vi "FeedbackDecode.vi"() -> ()   [LabVIEW 2020] (continued)
  T12 = cluster{"ExperimentDate":timestamp, "ImplantDate":timestamp, "CerebusFolder":string, "Experimenter":string, "PatientNumber":string, "DominantHand":string, "DeviceType":string, "DeviceSerial":string, "DeviceHemisphere":string, "DeviceRegion":string, "TaskType":string, "TaskComments":string, "RecordingComments":string, "GeneralObservations":string}
  T13 = typedef "FeedbackDecode_CogLoadClust.ctl" = cluster{"EEGTrigger":bool, "ConnectECG":bool, "TriggerECGwithTargets":bool, "SecondaryTask":bool, "MinTimeBetweenStimuli":dbl, "VariableTimeBetweenStimuli":dbl, "StimulusDuration":dbl, "RecordIMUwithTraining":bool, "ConnectIMU":bool}
  T14 = cluster{"[0]":u32, "[1]":u32, "[2]":u32, "[3]":u32}
  T15 = enum16{"---", "ReadMvnt", "WriteMvnt", "ReadEncode", "WriteEncode", "ReadDecode", "WriteDecode"}
  T16 = enum16{"Initialize", "Acquire Start", "Acquire Response", "Finalize"}
  T17 = enum8{"Enabled", "Disabled", "Disabled and Grayed Out"}
  T18 = enum16{"---", "Bakeoff11", "Bakeoff21", "Bakeoff31", "Bakeoff32", "LukeEmpty", "MPLEmpty", "MPLUnknown", "MPLBasic", "MPLTarg", "LukeBasic"}
  T19 = enum16{"Initialize", "Wait", "BuildInitStr", "BuildKalmanStr", "BuildStimStr", "BuildEMGStr", "GetEvent", "SendEvent", "ContIO", "LoadTrainFile", "CopyTraining", "Close"}
  T20 = cluster{"LV":cluster{"Name":string, "IP":string}, "ML":cluster{"Name":string, "IP":string}}
  T21 = enum32{"Invalid", "Standard", "Closed", "Hidden", "Minimized", "Maximized"}
  T22 = enum16{"open", "replace", "create", "open or create", "replace or create", "replace or create with confirmation"}
  T23 = enum16{"MSMS", "Bakeoff11", "Bakeoff21", "Bakeoff31", "Bakeoff32", "Bakeoff32_Ball", "Bakeoff32_Checkers", "Bakeoff32_Pen", "FragileBlock"}
  T24 = cluster{"MvntMat":dbl[][], "MvntName":string, "Tracking":enum8{"False", "True", "Mixed"}, "Radius":dbl}[]
  T25 = cluster{"Boolean 1":bool, "Boolean 2":bool, "Boolean 3":bool, "Boolean 4":bool, "Boolean 5":bool, "Boolean 6":bool, "Boolean 7":bool, "Boolean 8":bool, "Boolean 9":bool, "Boolean 10":bool, "Boolean 11":bool, "Boolean 12":bool, "Boolean 13":bool, "Boolean 14":bool, "Boolean 15":bool, "Boolean 16":bool, "Boolean 17":bool, "Boolean 18":bool, "Boolean 19":bool, "Boolean 20":bool, "Boolean 21":bool, "Boolean 22":bool, "Boolean 23":bool, "Boolean 24":bool, "Boolean 25":bool, "Boolean 26":bool, "Boolean 27":bool, "Boolean 28":bool, "Boolean 29":bool, "Boolean 30":bool, "Boolean 31":bool, "Boolean 32":bool, "Boolean 33":bool, "Boolean 34":bool, "Boolean 35":bool, "Boolean 36":bool, "Boolean 37":bool, "Boolean 38":bool, "Boolean 39":bool, "Boolean 40":bool, "Boolean 41":bool, "Boolean 42":bool, "Boolean 43":bool, "Boolean 44":bool, "Boolean 45":bool, "Boolean 46":bool, "Boolean 47":bool, "Boolean 48":bool, "Boolean 49":bool, "Boolean 50":bool, "Boolean 51":bool, "Boolean 52":bool, "Boolean 53":bool, "Boolean 54":bool, "Boolean 55":bool, "Boolean 56":bool, "Boolean 57":bool, "Boolean 58":bool, "Boolean 59":bool, "Boolean 60":bool, "Boolean 61":bool, "Boolean 62":bool, "Boolean 63":bool, "Boolean 64":bool, "Boolean 65":bool, "Boolean 66":bool, "Boolean 67":bool, "Boolean 68":bool, "Boolean 69":bool, "Boolean 70":bool, "Boolean 71":bool, "Boolean 72":bool, "Boolean 73":bool, "Boolean 74":bool, "Boolean 75":bool, "Boolean 76":bool, "Boolean 77":bool, "Boolean 78":bool, "Boolean 79":bool, "Boolean 80":bool, "Boolean 81":bool, "Boolean 82":bool, "Boolean 83":bool, "Boolean 84":bool, "Boolean 85":bool, "Boolean 86":bool, "Boolean 87":bool, "Boolean 88":bool, "Boolean 89":bool, "Boolean 90":bool, "Boolean 91":bool, "Boolean 92":bool, "Boolean 93":bool, "Boolean 94":bool, "Boolean 95":bool, "Boolean 96":bool, "Boolean 97":bool, "Boolean 98":bool, "Boolean 99":bool, "Boolean 100":bool}[]
  T26 = cluster{"[0]":dbl, "[1]":dbl, "[2]":dbl, "[3]":dbl, "[4]":dbl, "[5]":dbl, "[6]":dbl, "[7]":dbl, "[8]":dbl, "[9]":dbl, "[10]":dbl, "[11]":dbl}
  T27 = typedef "XDNodeRunTimeDep.lvlib/timing_clust.ctl" = cluster{"Expected End [f-1]":u64, "Actual End [f-1]":u64, "Finished Late? [f-1]":bool, "Expected End [i-1]":u64, "Actual End [i-1]":u64, "Finished Late? [i-1]":bool, "Expected Start [i]":u64, "Actual Start [i]":u64, "Expected Start [f]":u64, "Actual Start [f]":u64, "Source Name":string, "Structure Name":string, "Period":i64, "Deadline":i64, "Offset":i64, "Start":i64, "Priority":i32, "Timeout":i32, "Mode":T28, "Wakeup Reason":T29, "Error":errorcluster, "Source Type":string, "Secondary Source Type":string, "Global End Time":u64, "Global Start Time":u64, "Frame Duration":u64, "Iteration Duration":u64, "Assigned CPU":i32, "I/O Scan Engine Mode":u32}
  T28 = typedef "XDNodeRunTimeDep.lvlib/nitl_modes.ctl" = enum32{"No Change", "Process missed periods, maintain original phase", "Discard missed periods, maintain original phase", "Process missed periods, ignore original phase", "Discard missed periods, ignore original phase"}
  T29 = typedef "XDNodeRunTimeDep.lvlib/wakeup.ctl" = enum32{"Normal", "Aborted", "Asynchronous wakeup", "Timing source error", "Timed loop error", "Timeout"}
  T30 = enum16{"MSMS", "BakeOff1", "BakeOff2", "BakeOff3"}
  T31 = typedef "LVPositionTypeDef.ctl" = cluster{"Left":i32, "Top":i32}
  T32 = typedef "LVBoundsTypeDef.ctl" = cluster{"Width":u32, "Height":u32}
  T33 = cluster{cluster{"[0]":u32, "[1]":u32, "[2]":u32, "[3]":u32}, "HMSize":cluster{"NumCol":dbl, "NumRows":dbl}}
  T34 = cluster{"Left":i32, "Top":i32, "Width":u32, "Height":u32}
  T35 = cluster{"Name":string, "Type":string, "ID":string, "Num":string, "COM":dbl[], "Offset":dbl[], "RotationAxis":dbl[], "OrientationMatrix":dbl[][], "MinAngle":dbl, "MaxAngle":dbl, "InboardID":string, "InboardNum":string, "InboardCOM":dbl[], "OutboardID":string, "OutboardNum":string, "OutboardCOM":dbl[]}[]
  T36 = cluster{"ModelName":string, "Value":dbl[][], "CompNames":string[]}
  T37 = enum16{"Off", "Training", "Decode", "COB", "LEAP"}
  T38 = cluster{"ContMvntVal[0]":dbl, "ContMvntVal[1]":dbl, "ContMvntVal[2]":dbl, "ContMvntVal[3]":dbl, "ContMvntVal[4]":dbl, "ContMvntVal[5]":dbl, "ContMvntVal[6]":dbl, "ContMvntVal[7]":dbl, "ContMvntVal[8]":dbl, "ContMvntVal[9]":dbl, "ContMvntVal[10]":dbl, "ContMvntVal[11]":dbl}
  T39 = cluster{"ContTargetVal[0]":dbl, "ContTargetVal[1]":dbl, "ContTargetVal[2]":dbl, "ContTargetVal[3]":dbl, "ContTargetVal[4]":dbl, "ContTargetVal[5]":dbl, "ContTargetVal[6]":dbl, "ContTargetVal[7]":dbl, "ContTargetVal[8]":dbl, "ContTargetVal[9]":dbl, "ContTargetVal[10]":dbl, "ContTargetVal[11]":dbl}
  T40 = cluster{"LoopTimings":cluster{"MLCalcTime":dbl, "MLTotalTime":dbl}, "Kalman":cluster{"Thumb":dbl, "Index":dbl, "Middle":dbl, "Ring":dbl, "Little":dbl, "ThumbInt":dbl, "IndexInt":dbl, "RingInt":dbl, "LittleInt":dbl, "Wrist":dbl, "WristYaw":dbl, "WristRoll":dbl}, "Kinematics":cluster{"Thumb":dbl, "Index":dbl, "Middle":dbl, "Ring":dbl, "Little":dbl, "ThumbInt":dbl, "IndexInt":dbl, "RingInt":dbl, "LittleInt":dbl, "Wrist":dbl, "WristYaw":dbl, "WristRoll":dbl}, "ElectRates":dbl[], "SelWfs":dbl[][], "TrainCnt":dbl, "EMGPwr":dbl[], "SelData":cluster{dbl, dbl, "RasterOut":dbl[]}[], "SelRate":cluster{"CurIdx":dbl, dbl, "RasterOut":dbl[]}[], "SelKin":cluster{dbl, dbl, "RasterOut":dbl[]}[], "NIPTime":dbl, "VREID":i16, "StimWf":dbl[], "RawDecodeOutput":dbl[], "TASKA IR sensors":dbl[], "TASKA baro sensors":dbl[]}
  T41 = cluster{"Thumb":dbl, "Index":dbl, "Middle":dbl, "Ring":dbl, "Little":dbl, "ThumbInt":dbl, "IndexInt":dbl, "RingInt":dbl, "LittleInt":dbl, "Wrist":dbl, "WristYaw":dbl, "WristRoll":dbl}
  T42 = cluster{"Delay":dbl, "Rise":dbl, "Hold":dbl, "Trial":dbl}
  T43 = enum16{"Position", "Latching", "Leaky", "Velocity"}[]
  T44 = enum16{"Standard", "Mean", "Refit", "LinSVReg", "NonLinSVReg", "PCA", "DWPRR", "AdaptKF", "NN", "NN_python", "AdaptKF2", "KF_Short_Goal"}
  T45 = typedef "LVPoint32TypeDef.ctl" = cluster{"Horizontal":i32, "Vertical":i32}
  T46 = cluster{"KGain":sgl[][], "KMvnts":cluster{"Thumb":bool, "Index":bool, "Middle":bool, "Ring":bool, "Little":bool, "ThumbInt":bool, "IndexInt":bool, "RingInt":bool, "LittleInt":bool, "WristPitch":bool, "WristYaw":bool, "WristRoll":bool}, "KThresh":sgl[][], "CtrlMode":enum16{"Position", "Latching", "Leaky", "Velocity"}[], "CtrlSpd":sgl[]}
  T47 = enum16{"RMS Single", "RMS All", "RMS Auto", "Volt Single", "Volt All"}
  T48 = cluster{"[0]":bool, "[1]":bool, "[2]":bool, "[3]":bool, "[4]":bool, "[5]":bool, "[6]":bool, "[7]":bool, "[8]":bool, "[9]":bool, "[10]":bool, "[11]":bool, "[12]":bool, "[13]":bool, "[14]":bool, "[15]":bool, "[16]":bool, "[17]":bool, "[18]":bool, "[19]":bool, "[20]":bool, "[21]":bool, "[22]":bool, "[23]":bool, "[24]":bool, "[25]":bool, "[26]":bool, "[27]":bool, "[28]":bool, "[29]":bool, "[30]":bool, "[31]":bool, "[32]":bool, "[33]":bool, "[34]":bool, "[35]":bool, "[36]":bool, "[37]":bool, "[38]":bool, "[39]":bool, "[40]":bool, "[41]":bool, "[42]":bool, "[43]":bool, "[44]":bool, "[45]":bool, "[46]":bool, "[47]":bool, "[48]":bool, "[49]":bool, "[50]":bool, "[51]":bool, "[52]":bool, "[53]":bool, "[54]":bool, "[55]":bool, "[56]":bool, "[57]":bool, "[58]":bool, "[59]":bool, "[60]":bool, "[61]":bool, "[62]":bool, "[63]":bool, "[64]":bool, "[65]":bool, "[66]":bool, "[67]":bool, "[68]":bool, "[69]":bool, "[70]":bool, "[71]":bool, "[72]":bool, "[73]":bool, "[74]":bool, "[75]":bool, "[76]":bool, "[77]":bool, "[78]":bool, "[79]":bool, "[80]":bool, "[81]":bool, "[82]":bool, "[83]":bool, "[84]":bool, "[85]":bool, "[86]":bool, "[87]":bool, "[88]":bool, "[89]":bool, "[90]":bool, "[91]":bool, "[92]":bool, "[93]":bool, "[94]":bool, "[95]":bool, "[96]":bool, "[97]":bool, "[98]":bool, "[99]":bool}
  T49 = cluster{"[0]":bool, "[1]":bool, "[2]":bool, "[3]":bool, "[4]":bool, "[5]":bool, "[6]":bool, "[7]":bool, "[8]":bool, "[9]":bool, "[10]":bool, "[11]":bool, "[12]":bool, "[13]":bool, "[14]":bool, "[15]":bool, "[16]":bool, "[17]":bool, "[18]":bool, "[19]":bool, "[20]":bool, "[21]":bool, "[22]":bool, "[23]":bool, "[24]":bool, "[25]":bool, "[26]":bool, "[27]":bool, "[28]":bool, "[29]":bool, "[30]":bool, "[31]":bool, "[32]":bool, "[33]":bool, "[34]":bool, "[35]":bool, "[36]":bool, "[37]":bool, "[38]":bool, "[39]":bool, "[40]":bool, "[41]":bool, "[42]":bool, "[43]":bool, "[44]":bool, "[45]":bool, "[46]":bool, "[47]":bool, "[48]":bool, "[49]":bool, "[50]":bool, "[51]":bool, "[52]":bool, "[53]":bool, "[54]":bool, "[55]":bool, "[56]":bool, "[57]":bool, "[58]":bool, "[59]":bool, "[60]":bool, "[61]":bool, "[62]":bool, "[63]":bool, "[64]":bool, "[65]":bool, "[66]":bool, "[67]":bool, "[68]":bool, "[69]":bool, "[70]":bool, "[71]":bool, "[72]":bool, "[73]":bool, "[74]":bool, "[75]":bool, "[76]":bool, "[77]":bool, "[78]":bool, "[79]":bool}
  T50 = enum16{"Position", "Latching", "Leaky", "Velocity"}
  T51 = cluster{"Shift":bool, "Ctrl":bool, "Alt":bool, "Cmd":bool, "Opt":bool}
  T52 = cluster{"Region":bool, "Receptor":bool, "Electrode":bool, "Min Amp":bool, "Max Amp":bool, "Min Freq":bool, "Max Freq":bool, "Duration":bool}
  T53 = typedef "eventvkey.ctl" = enum16{"ASCII", "Enter", "Return", "Shift", "Ctrl", "Alt", "Cmd", "Opt", "Caps", "NumLock", "Clear", "Break", "Up", "Down", "Left", "Right", "Insert", "Delete", "Home", "End", "PageUp", "PageDown", "Escape", "Help", "Pause", "ScrollLock", "F1", "F2", "F3", "F4", "F5", "F6", "F7", "F8", "F9", "F10", "F11", "F12", "F13", "F14", "F15", "F16", "F17", "F18", "F19", "F20", "F21", "F22", "F23", "F24", "Play", "VolumeUp", "VolumeDown", "Mute", "Two Byte Char"}
  T54 = cluster{"Boolean 1":bool, "Boolean 2":bool, "Boolean 3":bool, "Boolean 4":bool, "Boolean 5":bool, "Boolean 6":bool, "Boolean 7":bool, "Boolean 8":bool, "Boolean 9":bool, "Boolean 10":bool, "Boolean 11":bool, "Boolean 12":bool, "Boolean 13":bool, "Boolean 14":bool, "Boolean 15":bool, "Boolean 16":bool, "Boolean 17":bool, "Boolean 18":bool, "Boolean 19":bool, "Boolean 20":bool, "Boolean 21":bool, "Boolean 22":bool, "Boolean 23":bool, "Boolean 24":bool, "Boolean 25":bool, "Boolean 26":bool, "Boolean 27":bool, "Boolean 28":bool, "Boolean 29":bool, "Boolean 30":bool, "Boolean 31":bool, "Boolean 32":bool, "Boolean 33":bool, "Boolean 34":bool, "Boolean 35":bool, "Boolean 36":bool, "Boolean 37":bool, "Boolean 38":bool, "Boolean 39":bool, "Boolean 40":bool, "Boolean 41":bool, "Boolean 42":bool, "Boolean 43":bool, "Boolean 44":bool, "Boolean 45":bool, "Boolean 46":bool, "Boolean 47":bool, "Boolean 48":bool, "Boolean 49":bool, "Boolean 50":bool, "Boolean 51":bool, "Boolean 52":bool, "Boolean 53":bool, "Boolean 54":bool, "Boolean 55":bool, "Boolean 56":bool, "Boolean 57":bool, "Boolean 58":bool, "Boolean 59":bool, "Boolean 60":bool, "Boolean 61":bool, "Boolean 62":bool, "Boolean 63":bool, "Boolean 64":bool, "Boolean 65":bool, "Boolean 66":bool, "Boolean 67":bool, "Boolean 68":bool, "Boolean 69":bool, "Boolean 70":bool, "Boolean 71":bool, "Boolean 72":bool, "Boolean 73":bool, "Boolean 74":bool, "Boolean 75":bool, "Boolean 76":bool, "Boolean 77":bool, "Boolean 78":bool, "Boolean 79":bool, "Boolean 80":bool, "Boolean 81":bool, "Boolean 82":bool, "Boolean 83":bool, "Boolean 84":bool, "Boolean 85":bool, "Boolean 86":bool, "Boolean 87":bool, "Boolean 88":bool, "Boolean 89":bool, "Boolean 90":bool, "Boolean 91":bool, "Boolean 92":bool, "Boolean 93":bool, "Boolean 94":bool, "Boolean 95":bool, "Boolean 96":bool, "Boolean 97":bool, "Boolean 98":bool, "Boolean 99":bool, "Boolean 100":bool}
  T55 = cluster{"[0]":bool, "[1]":bool, "[2]":bool, "[3]":bool, "[4]":bool, "[5]":bool, "[6]":bool, "[7]":bool, "[8]":bool, "[9]":bool, "[10]":bool, "[11]":bool, "[12]":bool, "[13]":bool, "[14]":bool, "[15]":bool, "[16]":bool, "[17]":bool, "[18]":bool, "[19]":bool, "[20]":bool, "[21]":bool, "[22]":bool, "[23]":bool, "[24]":bool, "[25]":bool, "[26]":bool, "[27]":bool, "[28]":bool, "[29]":bool, "[30]":bool, "[31]":bool, "[32]":bool, "[33]":bool, "[34]":bool, "[35]":bool, "[36]":bool, "[37]":bool, "[38]":bool, "[39]":bool, "[40]":bool, "[41]":bool, "[42]":bool, "[43]":bool, "[44]":bool, "[45]":bool, "[46]":bool, "[47]":bool, "[48]":bool, "[49]":bool, "[50]":bool, "[51]":bool, "[52]":bool, "[53]":bool, "[54]":bool, "[55]":bool, "[56]":bool, "[57]":bool, "[58]":bool, "[59]":bool, "[60]":bool, "[61]":bool, "[62]":bool, "[63]":bool, "[64]":bool, "[65]":bool, "[66]":bool, "[67]":bool, "[68]":bool, "[69]":bool, "[70]":bool, "[71]":bool, "[72]":bool, "[73]":bool, "[74]":bool, "[75]":bool, "[76]":bool, "[77]":bool, "[78]":bool, "[79]":bool, "[80]":bool, "[81]":bool, "[82]":bool, "[83]":bool, "[84]":bool, "[85]":bool, "[86]":bool, "[87]":bool, "[88]":bool, "[89]":bool, "[90]":bool, "[91]":bool, "[92]":bool, "[93]":bool, "[94]":bool, "[95]":bool, "[96]":bool, "[97]":bool, "[98]":bool, "[99]":bool}[]
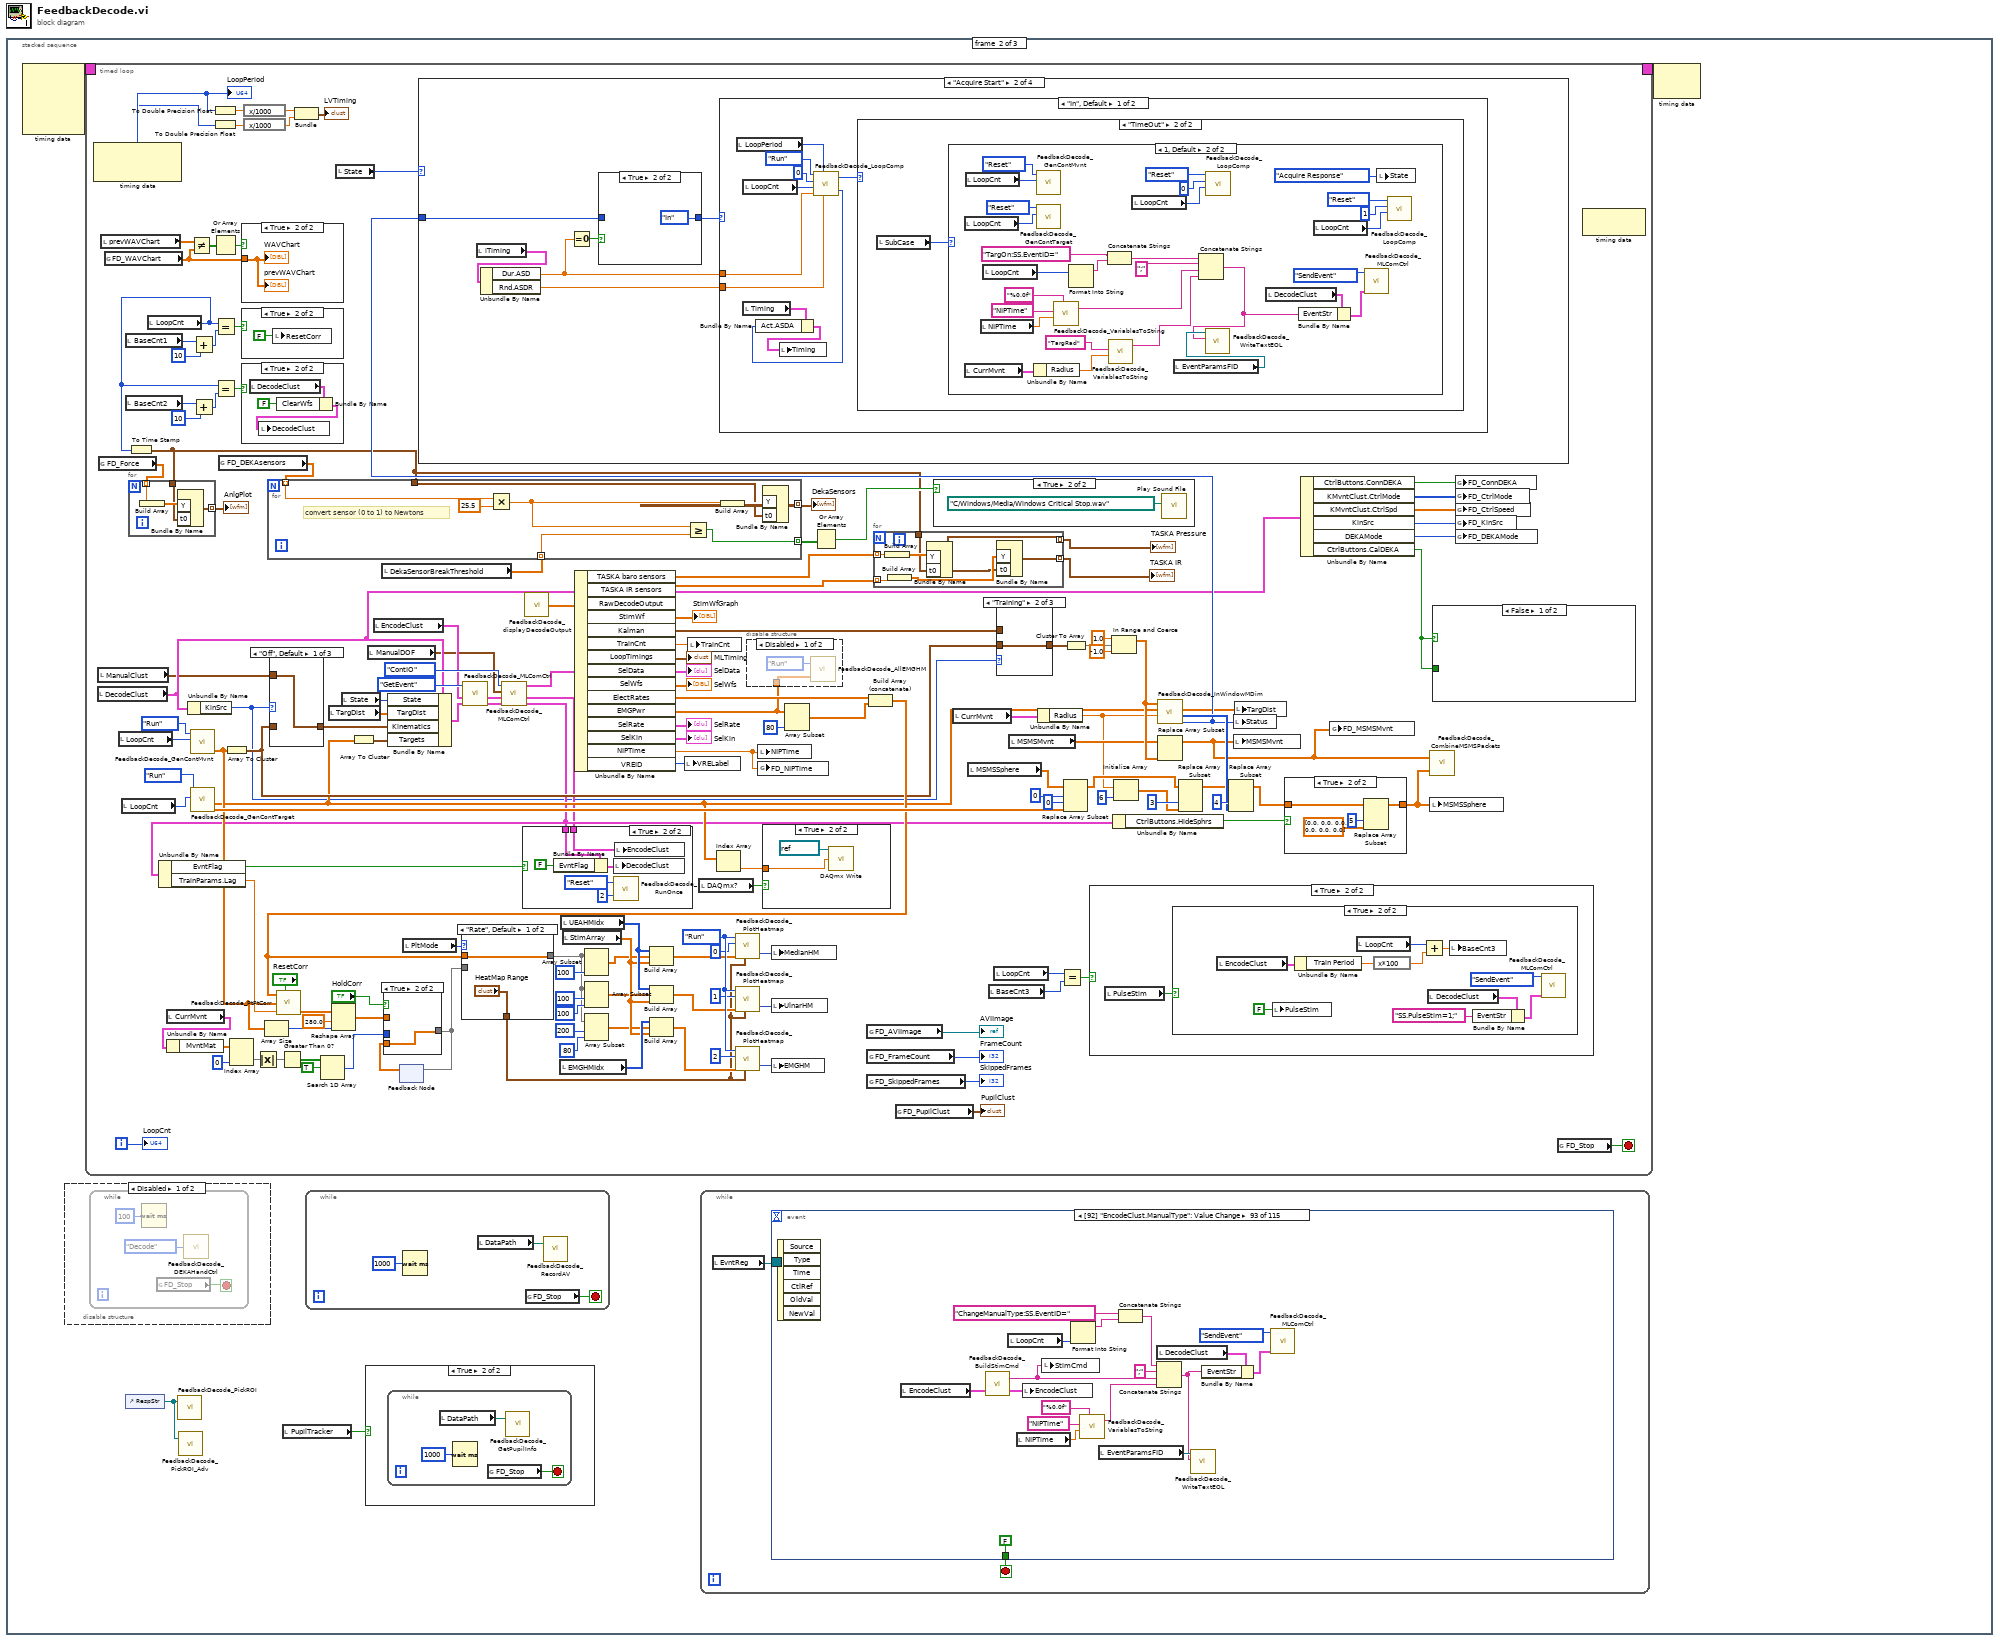
[diagram p0: block diagram]
diagram:
  n1 = stacked-sequence {
    frame #0 {
      n2 = stacked-sequence {
        frame #0 {
          w45 = FALSE ("Finished")
          w52 = 0.0  # MvntEvnt
          w68 = u64 0 ("BaseCnt1")
          w155 = enum16{"Initialize", "Reset", "Run"}."Initialize" ("Mode")
          w141 = "" ("TrialTypeStr")
          w122 = path "Z:/Shared drives/CNI/General/Databases/PatientDatabase.udl" ("DatabaseUDL")
          # "Is shared enabled?"
          # "TASKA"
          # "for analog sensors"
          n3 = local write "TASKASharedControlBeta"(0.0 ("TASKASharedControlBeta")) -> ()
          n4 = local write "Beta Mode"("Fixed" ("Beta Mode")) -> ()
          n5 = local write "Computer Goal"("Close" ("Computer Goal")) -> ()
          n6 = local write "TASKA Shared Control"(FALSE ("TASKA Shared Control")) -> ()
          n7 = property on="MedianHM" class="Pict"() -> ("Position"=w119:T31, "Draw Area Size"=w118:T32)  [unwired: 2 in, 2 out]
          n8 = property on="UlnarHM" class="Pict"() -> ("Position"=w114:T31, "Draw Area Size"=w115:T32)  [unwired: 2 in, 2 out]
          n9 = property on="EMGHM" class="Pict"() -> ("Position"=w100:T31, "Draw Area Size"=w99:T32)  [unwired: 2 in, 2 out]
          n10 = Initialize Array(0.0 ("element"), 496 ("dimension size")) -> (w54:dbl[])
          n11 = Cluster To Array(cluster=w119) -> (array=w148:i32[])
          n12 = Cluster To Array(cluster=w118) -> (array=w149:u32[])
          n13 = Cluster To Array(cluster=w114) -> (array=w113:i32[])
          n14 = Cluster To Array(cluster=w115) -> (array=w112:u32[])
          n15 = Cluster To Array(cluster=w100) -> (array=w101:i32[])
          n16 = Cluster To Array(cluster=w99) -> (array=w102:u32[])
          n17 = call "FeedbackDecode_AllEMGHM.vi"("Intensities"=w54, "Mode"=enum16{"Initialize", "Run"}."Initialize") -> ()  [unwired: 2 in]
          n18 = property on="Finished" class="Bool (strict)"("DisabledEnum"=T17."Disabled and Grayed Out" ("Disabled"), "Value"=w45, "Blinking"=w45) -> ()  [unwired: 2 in, 2 out]
          n19 = Build Array (concatenate)(w148, w149) -> (w150:u32[])
          n20 = Build Array (concatenate)(w113, w112) -> (w111:u32[])
          n21 = Build Array (concatenate)(w101, w102) -> (w103:u32[])
          n22 = mathscript code="GridArray = reshape(rot90(reshape(1:100,10,10),-1),1,100);"() -> ("GridArray"=→"UEAHMIdx":i32[])  [unwired: 1 in, 1 out]
          n23 = property on="ParamsTable" class="Arr (strict)"() -> ("Index Values"=w81:u32[], "Left"=w73:i32, "Width"=w72:u32)  [unwired: 2 in, 2 out]
          n24 = Array To Cluster(array=w150) -> (cluster=w151:T14)
          "MedianPos" <- w151
          n25 = Array To Cluster(array=w111) -> (cluster=w107:T14)
          "UlnarPos" <- w107
          n26 = Array To Cluster(array=w103) -> (cluster=w98:T14)
          "EMGPos" <- w98
          n27 = for {
            N: 2 -> [_]
            tunnel: [w180] -> w43 mode=indexing
            i -> [w179]
            n28 = case shown="0, Default" w179 {
              tunnel: [w181 w185] -> w180
              frame 0, Default {
                n29 = vi-ref "FeedbackDecode_PickROI.vi"() -> (w184:refnum<vi>)
                n30 = invoke class="VI" method="FP.Open"(reference=w184, "Activate"=TRUE ("Activate?"), "State"=T21."Hidden") -> (reference out=w181:refnum<vi>)  [unwired: 2 in, 4 out]
              }
              frame 1 {
                n31 = vi-ref "FeedbackDecode_PickROI_Adv.vi"() -> (w188:refnum<vi>)
                n32 = invoke class="VI" method="FP.Open"(reference=w188, "Activate"=TRUE ("Activate?"), "State"=T21."Hidden") -> (reference out=w185:refnum<vi>)  [unwired: 2 in, 4 out]
              }
            }
          }
          "RespRefArray" <- w43
          n33 = stacked-sequence {
            frame #0 {
              w171 = FALSE ("TASKA Reset Success")
              n34 = local write "TASKA Reset Success"(w171) -> ()
              n35 = local write "TASKA Reset Break"(w171) -> ()
              n36 = local write "TASKA Timer"(w171) -> ()
            }
            frame #1 {
              n37 = property on="TASKA Timer" class="Bool (strict)"("DisabledEnum"=T17."Enabled" ("Disabled")) -> ()  [unwired: 2 in, 2 out]
            }
          }
          n38 = Bundle(w151, "HMSize"="HMSize") -> (w152:T33)  [unwired: 1 in]
          n39 = Bundle(w107, "HMSize"="HMSize") -> (w108:T33)  [unwired: 1 in]
          n40 = Bundle(w98, "HMSize"="HMSize") -> (w106:T33)  [unwired: 1 in]
          n41 = call "FeedbackDecode_PlotHeatmap.vi"("InitCluster"=w152, "Instance"=0, "Mode"=enum16{"Initialize", "Run", "Mouse"}."Initialize") -> ("Pic"=→"MedianHM":picture, "CurrPos"=w92:i32)  [unwired: 3 in]
          "SelElect" <- w92
          n42 = call "FeedbackDecode_PlotHeatmap.vi"("InitCluster"=w108, "Instance"=1, "Mode"=enum16{"Initialize", "Run", "Mouse"}."Initialize") -> ("Pic"=→"UlnarHM":picture)  [unwired: 3 in, 1 out]
          n43 = call "FeedbackDecode_PlotHeatmap.vi"("InitCluster"=w106, "Instance"=2, "Mode"=enum16{"Initialize", "Run", "Mouse"}."Initialize") -> ("Pic"=→"EMGHM":picture)  [unwired: 3 in, 1 out]
          n44 = property on="Sel" class="Arr (strict)"("Index Values"=w81) -> ()  [unwired: 2 in, 2 out]
          n45 = Bundle("Left"=w73, "Width"=w72) -> (→"ParamsTableLoc":cluster{"Left":i32, "Width":u32})  [unwired: 1 in]
          n46 = disable-structure shown="Disabled" {
            frame Disabled {
              n47 = vi-ref "FeedbackDecode_MSMS2DEKA.vi"() -> (w178:refnum<vi>)
              n48 = invoke class="VI" method="FP.Open"(reference=w178, "Activate"=FALSE ("Activate?"), "State"=T21."Minimized") -> ()  [unwired: 2 in, 5 out]
            }
            frame Enabled {
            }
          }
          n49 = property class="VI"() -> ("Name"=→"TaskType":string)  [unwired: 2 in, 2 out]
          n50 = property on="KUEA" class="Clust (strict)"() -> ("Left"=w166:i32, "Top"=w165:i32, "Width"=w164:u32, "Height"=w163:u32)  [unwired: 2 in, 2 out]
          n51 = for {
            N: 80 -> [_]
            tunnel: [w192] -> w96 mode=indexing
            i -> [w193]
            n52 = Increment(x=w193) -> (x+1=w192:i32)
          }
          "EMGHMIdx" <- w96
          n53 = Initialize Array(0.0 ("element"), 100 ("dimension size")) -> (→"StimArray":dbl[])
          n54 = Bundle("Left"=w166, "Top"=w165, "Width"=w164, "Height"=w163) -> (w162:T34)  [unwired: 1 in]
          "HoverPicPos" <- w162
          n55 = call <vilib>:"Application Directory.vi"() -> ("Application Directory"=w2:path)
          n56 = call <vilib>:"Check if File or Folder Exists.vi"("path"=path "D:/") -> ("file or folder exists?"=w21:bool)  [unwired: 8 in, 2 out]
          n57 = vi-ref "FeedbackDecode_PlaySound.vi"() -> (w157:refnum<vi>)
          n58 = disable-structure shown="Disabled" {
            frame Disabled {
              n59 = vi-ref "FeedbackDecode_AllEMGHM.vi"() -> (w189:refnum<vi>)
              n60 = invoke class="VI" method="FP.Open"(reference=w189, "Activate"=FALSE ("Activate?"), "State"=T21."Minimized") -> ()  [unwired: 2 in, 5 out]
            }
            frame Enabled {
            }
          }
          n61 = Build Path(base path=w2, name or relative path="resources") -> (appended path=w1:path)
          "ResourcesDir" <- w1
          n62 = Build Path(base path=w2, name or relative path="build") -> (appended path=w13:path)
          "BuildDir" <- w13
          n63 = call "FeedbackDecode_HoverElect.vi"("Border"=2.0, "PicPos"=w162, "Mode"=enum16{"Initialize", "Run"}."Initialize") -> ("Elect"=w143:i32)  [unwired: 3 in, 1 out]
          n64 = property class="VI"(reference=w157) -> ("Name"=w156:string)  [unwired: 1 in, 2 out]
          n65 = Select(t=path "D:/FeedbackDecode", s=w21, f=path "C:/Data/FeedbackDecode" ("path")) -> (s? t:f=w17:path)
          "DataDir" <- w17
          n66 = global write "FeedbackDecode_Globals.vi" "FD_ResourcesDir"(w1) -> ()
          n67 = Unbundle By Name("DecodeClust") -> ("NumComp"=w26:enum16{"1 Computer", "2 Computers"})
          n68 = Path To String(path=w13) -> (string=w15:string)
          n69 = Path To String(path=w17) -> (string=w19:string)
          n70 = Unbundle By Name("MvntBuilder") -> ("Mode"=w36:enum16{"Selected", "Block", "Random"}, "NTrials"=w39:dbl, "MvntList"=w40:T24)
          n71 = property on="MvntList" class="Arr (strict)"() -> ("Index Values"=w42:u32[])  [unwired: 2 in, 2 out]
          n72 = Open VI Reference(type specifier VI Refnum (for type only)=refnum<vi> refnum ("application reference (local)"), vi path=w156, options=128) -> (vi reference=→"PSRef":refnum<vi>)  [unwired: 3 in, 1 out]
          n73 = Unbundle By Name("MvntBuilder") -> ("TargParams.Radius"=w87:dbl)
          n74 = Search and Replace String(input string=w15, search string=":", replace string="@" ("replace string (\"\")")) -> (result string=w12:string)  [unwired: 5 in, 3 out]
          n75 = Search and Replace String(input string=w19, search string=":", replace string="@" ("replace string (\"\")")) -> (result string=w11:string)  [unwired: 5 in, 3 out]
          n76 = case shown="\"1 Computer\"" w26 {
            tunnel: [T20 {"LV"={"Name"="PNILABVIEW", "IP"="155.100.90.215"}, "ML"={"Name"="PNIMATLAB", "IP"="155.100.90.185"}} ("CompID") T20 {"LV"={"Name"="PNILABVIEW", "IP"="127.0.0.1"}, "ML"={"Name"="PNIMATLAB", "IP"="127.0.0.2"}} ("CompID")] -> w25
            frame "2 Computers", Default {
            }
            frame "1 Computer" {
            }
          }
          n77 = Array Size(array=w40) -> (size(s)=w41:i32)
          n78 = Index Array(array=w42) -> (element=w38:u32)  [unwired: 1 in]
          n79 = call "FeedbackDecode_GenRandBlockIdxs2.vi"("Mode"=w36, "Reset"=TRUE, "NumTrials"=w39, "NumIdxs"=w41, "CurrIdx"=w38) -> ("Perc"=w34:dbl)  [unwired: 1 out]
          n80 = Initialize Array(0.0 ("element"), 2 ("dimension size"), 12 ("dimension size")) -> (w77:dbl[][])
          n81 = Bundle By Name(cluster="MvntBuilder", "PercTrials"=w34) -> (w33:T6)
          n82 = call "FeedbackDecode_RunOnce.vi"("Instance"=0, "Mode"=enum16{"Reset", "Run"}."Reset") -> ()  [unwired: 1 out]
          n83 = Bundle By Name(cluster="DecodeClust", "BuildDir"=w12, "DataDir"=w11, "TrainParams.TargRad"=w87, "DataFolder"="00000000-000000", "SelElect"=w92, "CompID"=w25, "HoverElect"=w143, "KinSrc"=enum16{"Off", "Training", "Decode", "COB"}."Off", "TrialCnt"=w77, "KDFFile"="") -> (w84:T5)
          n84 = Unbundle By Name(w25) -> ("LV.IP"=→"LVIP":string, "ML.IP"=→"MLIP":string)
          n85 = local write "MvntBuilder"(w33) -> ()
          n86 = call "FeedbackDecode_RunOnce.vi"("Instance"=1, "Mode"=enum16{"Reset", "Run"}."Reset") -> ()  [unwired: 1 out]
          n87 = call "FeedbackDecode_RunOnce.vi"("Instance"=2, "Mode"=enum16{"Reset", "Run"}."Reset") -> ()  [unwired: 1 out]
          n88 = global write "FeedbackDecode_Globals.vi" "FD_Stop"(FALSE ("EnablePtCtrl")) -> ()
          n89 = call "FeedbackDecode_MLComCtrl.vi"("CognitiveLoadIn"="CognitiveLoad", "DecodeClustIn"=w84, "EncodeClustIn"="EncodeClust", "Mode"=T19."Initialize") -> ("DecodeClustOut"=w32:T5, "EncodeClustOut"=w82:T9, "CognitiveLoadOut"=w4:T13)  [unwired: 4 in, 1 out]
          n90 = property class="DAQmx System"() -> ("DevNames"=w30:tag[])  [unwired: 2 in, 2 out]
          n91 = Unbundle By Name(w32) -> ("RasterWin"=w88:dbl)
          n92 = Unbundle By Name(w32) -> ("*Prosthesis"=w58:enum16{"MaleRight", "MaleLeft"})
          n93 = Create User Event(user event datatype=w52) -> (user event=w51:refnum<user-event>)  [unwired: 1 in, 1 out]
          "MvntEvnt" <- w51
          n94 = local write "EncodeClust"(w82) -> ()
          n95 = local write "CognitiveLoad"(w4) -> ()
          n96 = local write "DecodeClust"(w32) -> ()
          n97 = register-events(w51) -> (reference out=→"EvntReg":refnum<event-registration>)  [unwired: 2 in, 1 out]
          n98 = Divide(x=w88, y=0.033) -> (x/y=w85:dbl)
          n99 = Empty Array?(array=w30) -> (empty?=w29:bool)
          n100 = Format Into String(w58) -> (resulting string=w135:string)  [unwired: 3 in, 1 out]
          n101 = Multiply(x=2.0, y=w85) -> (x*y=w86:dbl)
          n102 = Not(x=w29) -> (.not. x?=→"DAQmx?":bool)
          n103 = property on="SelData" class="WFGraph (strict)"("XScale.Maximum"=w86) -> ()  [unwired: 2 in, 2 out]
          n104 = property on="SelRate" class="WFGraph (strict)"("XScale.Maximum"=w85) -> ()  [unwired: 2 in, 2 out]
          n105 = property on="SelKin" class="WFGraph (strict)"("XScale.Maximum"=w85) -> ()  [unwired: 2 in, 2 out]
          n106 = case shown="False" w29 {
            frame False {
              n107 = call <vilib>:"DAQmx Start Task.vi"("task/channels in"=refnum<k21> "AO0") -> ()  [unwired: 13 in, 2 out]
            }
            frame True {
            }
          }
          n108 = Concatenate Strings("Z:\\Shared drives\\CNI\\General\\MSMS\\Scenarios\\", w135, "\\Model\\Prostheses\\prosthesis.xml") -> (w137:string)
          n109 = String To Path(string=w137) -> (path=w138:path)
          "XMLFile" <- w138
          n110 = call "FeedbackDecode_ParseMSMSXML.vi"("XMLFile"=w138) -> ("ComponentArray"=w132:T35)
          n111 = call "FeedbackDecode_UpdateDatabase.vi"("CallType"=enum16{"Initialize", "Save", "Load"}."Initialize", "DatabaseUDL"=w122) -> ("ExperimentDatesSorted"=w124:string[])  [unwired: 2 in, 2 out]
          n112 = call "FeedbackDecode_LoadMSMSParams.vi"("XMLFile"=w138) -> ("ModelParams"=w133:T36)  [unwired: 1 in]
          n113 = call "FeedbackDecode_SendMSMSPacket.vi"("CompArrayIn"=w132, "Mode"=enum16{"Initialize", "Run", "Close"}."Initialize") -> ()  [unwired: 5 in]
          n114 = property on="RecordSel" class="CmbBox"("Text.Text"="", "Strings[]"=w124) -> ()  [unwired: 2 in, 2 out]
          n115 = call "FeedbackDecode_BuildMSMSMvnt.vi"("CompArray"=w132, "ModelParams"=w133, "Mode"=enum16{"Initialize", "Run"}."Initialize") -> ()  [unwired: 4 in, 3 out]
          n116 = call "FeedbackDecode_GenContTarget.vi"("Mode"=w155) -> ()  [unwired: 5 in, 4 out]
          n117 = call "FeedbackDecode_GenContMvnt.vi"("Mode"=w155) -> ()  [unwired: 5 in, 3 out]
          n118 = call "FeedbackDecode_BuildMSMSSphere.vi"("CompArray"=w132, "ModelParams"=w133, "Mode"=enum16{"Initialize", "Run"}."Initialize") -> ()  [unwired: 4 in, 3 out]
          "State" <- T16."Initialize" ("Current State")
          "BaseCnt1" <- w68
          "TrialParameters" <- w141
          "DatabaseUDL" <- w122
          "TaskParameters" <- w141
          "Outcome" <- enum16{"---", "Success", "Failure"}."---" ("Outcome")
          "TrialArray" <- string[] [] ("TrialArray")
          "PrevIdx" <- 0.0 ("PrevIdx")
          "BaseCnt2" <- w68
          "TrainCnt" <- 0.0 ("TrainCnt")
          "Status" <- enum16{"In", "Out"}."Out" ("Status")
          "FileIO" <- T15."---" ("FileIO")
          "TargDist" <- dbl[] [0.0, 0.0, 0.0, 0.0, 0.0, 0.0] ("TargDist")
          "iTiming" <- "Timing"
          "NIPTime" <- 0.0 ("TrainCnt")
          "VRELabel" <- T18."---" ("VRELabel")
          "BaseCnt3" <- -inf
          "PulseStim" <- FALSE ("PulseStim")
          "RespStr" <- ""
          "StimCmd" <- ""
          "SelTog" <- FALSE ("SelTog")
          "StimTog" <- FALSE ("StimTog")
          "CurrMvnt" <- T1 {"MvntMat"=[], "MvntName"="", "Tracking"=enum."False", "Radius"=0.15} ("CurrMvnt")
        }
        frame #1 {
          # "Open Trellis if it is not already running"
          n119 = call <vilib>:"System Exec.vi"("command line"="powershell -inputformat none -command get-process -name Trellis") -> ("error out"=w242:errorcluster, "standard output"=w244:string)  [unwired: 7 in, 2 out]
          n120 = Empty String/Path?(string/path=w244) -> (empty?=w243:bool)
          n121 = case shown="True" w243 {
            tunnel: [w246 w248] -> w241
            tunnel: w242 -> [w246 w247]
            frame False {
            }
            frame True {
              n122 = Path To String(path=path "C:/Program Files (x86)/Ripple/Trellis/Apps/Trellis/bin/start_Trellis.bat") -> (string=w251:string)
              n123 = call <vilib>:"System Exec.vi"("wait until completion? (T)"=FALSE, "error in (no error)"=w247, "working directory"=path "C:/Program Files (x86)/Ripple/Trellis/Apps/Trellis/bin", "command line"=w251) -> ("error out"=w248:errorcluster)  [unwired: 4 in, 3 out]
            }
          }
          n124 = case shown="No Error" w241 {
            tunnel: w241 -> [_ w254]
            frame No Error {
              n125 = One Button Dialog(message="Load Trellis config file, enable appropriate channels for saving to disk, set file save directory to \"D:\\\", and make sure digital triggering is enabled.\n\nDigital Triggering...\nStart: Parallel (0x007F; 0x0011)\nStop: Parallel (0x007F; 0x0012) ") -> ()  [unwired: 1 in, 1 out]
            }
            frame Error {
              n126 = call <vilib>:"Simple Error Handler.vi"("error in (no error)"=w254) -> ()  [unwired: 4 in, 5 out]
            }
          }
        }
        frame #2 {
          n127 = call "FeedbackDecode_CheckPupilConnection.vi"() -> ("Connected?"=w255:bool)  [unwired: 1 in]
          "PupilTracker" <- w255
          n128 = case shown="True" w255 {
            frame False {
            }
            frame True {
              n129 = call <vilib>:"System Exec.vi"("command line"="powershell -inputformat none -command get-process -name pupil_capture") -> ("error out"=w257:errorcluster, "standard output"=w259:string)  [unwired: 7 in, 2 out]
              n130 = Empty String/Path?(string/path=w259) -> (empty?=w258:bool)
              n131 = case shown="True" w258 {
                tunnel: [w261 w263] -> w256
                tunnel: w257 -> [w261 w262]
                frame False {
                }
                frame True {
                  n132 = Path To String(path=path "C:/Program Files (x86)/Pupil-Labs/Pupil v2.6.19/Pupil Capture v2.6.19/pupil_capture.exe") -> (string=w265:string)
                  n133 = call <vilib>:"System Exec.vi"("wait until completion? (T)"=FALSE, "error in (no error)"=w262, "command line"=w265) -> ("error out"=w263:errorcluster)  [unwired: 5 in, 3 out]
                }
              }
              n134 = case shown="No Error" w256 {
                tunnel: w256 -> [_ w268]
                frame No Error {
                  n135 = One Button Dialog(message="Make sure eye tracker is plugged into usb and eye0 process is running in 3d mode with pupil detected. Set pupil remote port to 55555. \n\nIf not using eye tracker, unplug from usb and close pupil capture software.") -> ()  [unwired: 1 in, 1 out]
                }
                frame Error {
                  n136 = call <vilib>:"Simple Error Handler.vi"("error in (no error)"=w268) -> ()  [unwired: 4 in, 5 out]
                }
              }
            }
          }
        }
        frame #3 {
          # "Create data folder and start params txt files"
          n137 = Get Date/Time In Seconds() -> (seconds since 1Jan1904=w286:timestamp)
          "ExperimentDate" <- w286
          n138 = local read "DataDir"() -> (w274:path)
          n139 = Format Date/Time String(time format string (%c)="%Y%m%d-%H%M%S", seconds (now)=w286) -> (date/time string=w269:string)  [unwired: 1 in]
          n140 = Build Path(base path=w274, name or relative path=w269) -> (appended path=w273:path)
          n141 = call <vilib>:"Check if File or Folder Exists.vi"("path"=w273) -> ("error out"=w272:errorcluster, "file or folder exists?"=w270:bool, "dup path"=w271:path)  [unwired: 8 in]
          n142 = case shown="False" w270 {
            tunnel: [w290 w292] -> w276
            tunnel: [w289 w291] -> w277
            tunnel: w272 -> [w288 w291]
            tunnel: w271 -> [w287 w292]
            frame False {
              n143 = Create Folder(path (use dialog)=w287, error in=w288) -> (created path=w290:path, error out=w289:errorcluster)  [unwired: 1 in, 1 out]
            }
            frame True {
            }
          }
          "DataPath" <- w276
          n144 = local read "DecodeClust"() -> (w275:T5)
          n145 = Bundle By Name(cluster=w275, "DataFolder"=w269) -> (w284:T5)
          n146 = local write "DecodeClust"(w284) -> ()
          n147 = Concatenate Strings("EventParams_" ("name or relative path"), w269, ".txt" ("string")) -> (w278:string)
          n148 = Build Path(base path=w276, name or relative path=w278) -> (appended path=w282:path)
          n149 = Open/Create/Replace File(file path (use dialog)=w282, error in=w277, operation (0:open)=T22."replace or create") -> (refnum out=→"EventParamsFID":refnum<file>)  [unwired: 3 in, 2 out]
        }
        frame #4 {
          # "start matlab executable on remote computer"
          n150 = local read "DecodeClust"() -> (w295:T5)
          n151 = Unbundle By Name(w295) -> ("StartML"=w294:bool, "NumComp"=w293:enum16{"1 Computer", "2 Computers"})
          n152 = case shown="True" w294 {
            tunnel: w293 -> [_ w296]
            frame False {
            }
            frame True {
              n153 = case shown="\"1 Computer\", Default" w296 {
                frame "1 Computer", Default {
                  n154 = local read "BuildDir"() -> (w297:path)
                  n155 = call <vilib>:"System Exec.vi"("wait until completion? (T)"=FALSE, "working directory"=w297, "command line"="cmd /c FeedbackDecode.exe 127.0.0.1") -> ()  [unwired: 5 in, 4 out]
                }
                frame "2 Computers" {
                  n156 = local read "TaskType"() -> (w303:string)
                  n157 = Search and Replace String(input string=w303, search string=".vi", replace string=".exe" ("replace string (\"\")")) -> (result string=w304:string)  [unwired: 5 in, 3 out]
                  n158 = local read "MLIP"() -> (w302:string)
                  n159 = local read "LVIP"() -> (w301:string)
                  n160 = Build Path(base path=path "D:/RemoteRepo", name or relative path=w304) -> (appended path=w305:path)
                  n161 = call "FeedbackDecode_RunProgram_PSExec.vi"("ProgramInput"=w301, "Program"=w305, "ComputerName"=w302, "Mode"=enum16{"Start", "Stop"}."Start") -> ()  [unwired: 1 out]
                }
              }
            }
          }
        }
        frame #5 {
          # "Wait for matlab to startup"
          n162 = call "FeedbackDecode_MLComCtrl.vi"("Mode"=T19."Wait") -> ()  [unwired: 7 in, 4 out]
        }
        frame #6 {
          # "MP: Added CL here"
          # "Send initialization variables to matlab"
          n163 = local read "CognitiveLoad"() -> (w312:T13)
          n164 = local read "EncodeClust"() -> (w321:T9)
          n165 = local read "DecodeClust"() -> (w322:T5)
          n166 = call "FeedbackDecode_MLComCtrl.vi"("CognitiveLoadIn"=w312, "DecodeClustIn"=w322, "EncodeClustIn"=w321, "Mode"=T19."BuildInitStr") -> ("DecodeClustOut"=w318:T5, "EncodeClustOut"=w319:T9, "CognitiveLoadOut"=w311:T13)  [unwired: 4 in, 1 out]
          n167 = Unbundle By Name(w318) -> ("EventStr"=w316:string, "NumComp"=→"NumComp":enum16{"1 Computer", "2 Computers"})
          n168 = call "FeedbackDecode_MLComCtrl.vi"("CognitiveLoadIn"=w311, "DecodeClustIn"=w318, "EncodeClustIn"=w319, "Mode"=T19."SendEvent") -> ("DecodeClustOut"=w323:T5, "EncodeClustOut"=w320:T9, "CognitiveLoadOut"=w310:T13)  [unwired: 4 in, 1 out]
          n169 = Concatenate Strings("InitParameters:" ("string"), w316) -> (w314:string)
          n170 = local read "EventParamsFID"() -> (w317:refnum<file>)
          n171 = local write "CognitiveLoad"(w310) -> ()
          n172 = local write "EncodeClust"(w320) -> ()
          n173 = local write "DecodeClust"(w323) -> ()
          n174 = call "FeedbackDecode_WriteTextEOL.vi"("text"=w314, "refnum in"=w317) -> ()  [unwired: 8 in, 2 out]
        }
        frame #7 {
          # "wait for matlab"
          n175 = call "FeedbackDecode_MLComCtrl.vi"("Mode"=T19."Wait") -> ()  [unwired: 7 in, 4 out]
        }
      }
    }
    frame #1 {
      n176 = node-c288() -> (w330:T27)  [unwired: 4 in]
      n177 = disable-structure shown="Disabled" {
        frame Disabled {
          n178 = while {
            stop <- w335 stop-if-true
            n179 = Wait (ms)(milliseconds to wait=u32 100) -> ()  [unwired: 1 out]
            n180 = global read "FeedbackDecode_Globals.vi" "FD_Stop"() -> (w335:bool)
            n181 = call "FeedbackDecode_DEKAHandCtrl.vi"("RunMode"=enum16{"Manual", "Decode"}."Decode") -> ()  [unwired: 1 in]
          }
        }
        frame Enabled {
        }
      }
      n182 = timed-loop {
        timing: w330 -> [_]
        timing-out: [_] -> w329
        i -> [w3398]
        stop <- w3280 stop-if-true
        w3331 = enum16{"Initialize", "Run", "Mouse"}."Run" ("Mode")
        n183 = node-c288() -> (w3402:i64, w3399:i64)  [unwired: 1 in]
        "LoopPeriod" <- w3402
        n184 = local read "DecodeClust"() -> (w3289:T5)
        n185 = local read "ManualClust"() -> (w3284:T7)
        n186 = global read "FeedbackDecode_Globals.vi" "FD_Force"() -> (w3272:dbl[])
        n187 = local read "prevWAVChart"() -> (w3385:dbl[])
        n188 = global read "FeedbackDecode_Globals.vi" "FD_WAVChart"() -> (w3386:dbl[])
        n189 = local read "LoopCnt"() -> (w3383:u64)
        n190 = local read "LoopCnt"() -> (w3389:u64)
        n191 = local read "BaseCnt1"() -> (w3359:u64)
        n192 = local read "BaseCnt2"() -> (w3357:u64)
        n193 = local read "LoopCnt"() -> (w3270:u64)
        n194 = To Time Stamp(1:w3270) -> (0:w3259:timestamp)
        n195 = for {
          tunnel: w3272 -> [w3428] mode=indexing
          tunnel: [w3427] -> w3271 mode=indexing
          tunnel: w3259 -> [w3426]
          n196 = Build Array(w3428) -> (w3429:dbl[])
          n197 = Bundle By Name("Y"=w3429, "t0"=w3426) -> (w3427:waveform(dbl))  [unwired: 1 in]
        }
        "AnlgPlot" <- w3271
        n198 = local read "CurrMvnt"() -> (w3377:T1)
        n199 = Unbundle By Name(w3377) -> ("MvntMat"=w3376:dbl[][])
        n200 = Unbundle By Name(w3289) -> ("KinSrc"=w3287:T37)
        n201 = Not Equal?(x=w3385, y=w3386) -> (x != y?=w3387:bool[])
        n202 = call "FeedbackDecode_GenContMvnt.vi"("Mode"=enum16{"Initialize", "Reset", "Run"}."Run", "LoopCount"=w3383) -> ("ContMvntVal"=w3348:dbl[])  [unwired: 4 in, 2 out]
        n203 = call "FeedbackDecode_GenContTarget.vi"("LoopCount"=w3389, "Mode"=enum16{"Initialize", "Reset", "Run"}."Run") -> ("ContSphereVal"=w3392:dbl[][], "ContTargetVal"=w3302:dbl[])  [unwired: 4 in, 2 out]
        n204 = Add(x=w3359, y=u64 10) -> (x+y=w3361:u64)
        n205 = Add(x=w3357, y=u64 10) -> (x+y=w3355:u64)
        n206 = To Double Precision Float(number=w3402) -> (double precision float=w3401:dbl)
        n207 = To Double Precision Float(number=w3399) -> (double precision float=w3400:dbl)
        n208 = Or Array Elements(Boolean array=w3387) -> (logical OR=w3388:bool)
        n209 = Equal?(x=w3270, y=w3361) -> (x = y?=w3362:bool)
        n210 = Equal?(x=w3270, y=w3355) -> (x = y?=w3354:bool)
        n211 = global read "FeedbackDecode_Globals.vi" "FD_DEKAsensors"() -> (w3269:dbl[])
        n212 = Array To Cluster(array=w3348) -> (cluster=w3312:T38)
        n213 = Index Array(array=w3376, index (col)=0 ("disabled index (col)")) -> (element=w3374:dbl[])  [unwired: 1 in]
        n214 = case shown="True" w3388 {
          tunnel: w3386 -> [_ w3489]
          frame False {
          }
          frame True {
            "prevWAVChart" <- w3489
            "WAVChart" <- w3489
          }
        }
        n215 = case shown="True" w3362 {
          frame False {
          }
          frame True {
            n216 = local write "ResetCorr"(FALSE ("ResetCorr")) -> ()
          }
        }
        n217 = case shown="True" w3354 {
          frame False {
          }
          frame True {
            n218 = local read "DecodeClust"() -> (w3478:T5)
            n219 = Bundle By Name(cluster=w3478, "ClearWfs"=FALSE) -> (w3480:T5)
            n220 = local write "DecodeClust"(w3480) -> ()
          }
        }
        n221 = expression code="x/1000"(w3401) -> (w3404:dbl)
        n222 = expression code="x/1000"(w3400) -> (w3403:dbl)
        n223 = Absolute Value(x=w3374) -> (abs(x)=w3373:dbl[])
        n224 = Array Size(array=w3348) -> (size(s)=w3369:i32)
        n225 = case shown="\"Off\", Default" w3287 {
          tunnel: [w3486 w3487 w3488] -> w3380
          tunnel: w3312 -> [_ w3487 _]
          tunnel: w3284 -> [w3486 _ w3488]
          frame "Off", Default {
          }
          frame "Training" {
          }
          frame "COB" {
          }
        }
        n226 = Greater Than 0?(x=w3373) -> (x > 0?=w3372:bool[])
        n227 = Bundle(w3404, w3403) -> (→"LVTiming":cluster{dbl, dbl})  [unwired: 1 in]
        n228 = Search 1D Array(1D array=w3372, element=TRUE) -> (index of element=w3364:i32)  [unwired: 1 in]
        n229 = local read "TargDist"() -> (w3341:dbl[])
        n230 = local read "State"() -> (w3405:T16)
        n231 = local read "State"() -> (w3342:T16)
        n232 = Array To Cluster(array=w3302) -> (cluster=w3381:T39)
        n233 = local read "ManualDOF"() -> (w3283:T8)
        n234 = local read "EncodeClust"() -> (w3294:T9)
        n235 = local read "DekaSensorBreakThreshold"() -> (w3265:dbl[])
        n236 = for {
          tunnel: w3269 -> [w3418] mode=indexing
          tunnel: [w3422] -> w3268 mode=indexing
          tunnel: w3259 -> [w3421]
          tunnel: w3265 -> [w3420] mode=indexing
          tunnel: [w3419] -> w3264 mode=indexing
          # "convert sensor (0 to 1) to Newtons"
          n237 = Multiply(x=w3418, y=25.5) -> (x*y=w3416:dbl)
          n238 = Greater Or Equal?(x=w3416, y=w3420) -> (x >= y?=w3419:bool)
          n239 = Build Array(w3416) -> (w3423:dbl[])
          n240 = Bundle By Name("Y"=w3423, "t0"=w3421) -> (w3422:waveform(dbl))  [unwired: 1 in]
        }
        "DekaSensors" <- w3268
        n241 = Bundle By Name(cluster=w3289, "State"=w3342, "TargDist"=w3341, "Kinematics"=w3380, "Targets"=w3381) -> (w3343:T5)
        n242 = feedback #1() -> (w3363:dbl[])  [unwired: 1 in]
        n243 = local read "PltMode"() -> (w3339:enum16{"Rate", "Corr"})
        n244 = call "FeedbackDecode_MLComCtrl.vi"("DecodeClustIn"=w3343, "EncodeClustIn"=w3294, "Mode"=T19."GetEvent") -> ("DecodeClustOut"=w3297:T5, "EncodeClustOut"=w3296:T9)  [unwired: 5 in, 2 out]
        n245 = call "FeedbackDecode_MLComCtrl.vi"("DecodeClustIn"=w3297, "EncodeClustIn"=w3296, "ManualDOF"=w3283, "Mode"=T19."ContIO") -> ("DecodeClustOut"=w3295:T5, "EncodeClustOut"=w3293:T9, "MLClust"=w3382:T40)  [unwired: 4 in, 1 out]
        n246 = Unbundle By Name(w3295) -> ("EvntFlag"=w3313:bool, "TrainParams.Lag"=w3368:dbl)
        n247 = case shown="True" w3313 {
          tunnel: w3295 -> [_ w3471]
          tunnel: w3293 -> [_ w3470]
          frame False {
          }
          frame True {
            n248 = Bundle By Name(cluster=w3471, "EvntFlag"=FALSE) -> (w3472:T5)
            n249 = local write "DecodeClust"(w3472) -> ()
            n250 = call "FeedbackDecode_RunOnce.vi"("Instance"=2, "Mode"=enum16{"Reset", "Run"}."Reset") -> ()  [unwired: 1 out]
            n251 = local write "EncodeClust"(w3470) -> ()
          }
        }
        n252 = local read "EMGHMIdx"() -> (w3323:i32[])
        n253 = local read "UEAHMIdx"() -> (w3327:i32[])
        n254 = local read "StimArray"() -> (w3322:dbl[])
        n255 = Unbundle By Name(w3382) -> ("TASKA baro sensors"=w3258:dbl[], "TASKA IR sensors"=w3257:dbl[], "RawDecodeOutput"=w3267:dbl[], "StimWf"=→"StimWfGraph":dbl[], "Kalman"=w3311:T41, "TrainCnt"=w3347:dbl, "LoopTimings"=→"MLTiming":cluster{"MLCalcTime":dbl, "MLTotalTime":dbl}, "SelData"=→"SelData":cluster{dbl, dbl, "RasterOut":dbl[]}[], "SelWfs"=→"SelWfs":dbl[][], "ElectRates"=w3340:dbl[], "EMGPwr"=w3276:dbl[], "SelRate"=→"SelRate":cluster{"CurIdx":dbl, dbl, "RasterOut":dbl[]}[], "SelKin"=→"SelKin":cluster{dbl, dbl, "RasterOut":dbl[]}[], "NIPTime"=w3274:dbl, "VREID"=w3292:i16)
        n256 = call "FeedbackDecode_displayDecodeOutput.vi"("Input"=w3267) -> ()
        n257 = local write "VRELabel"(w3292) -> ()
        n258 = local write "TrainCnt"(w3347) -> ()
        n259 = local read "DAQmx?"() -> (w3261:bool)
        n260 = Index Array(array=w3302) -> (element=w3301:dbl)  [unwired: 1 in]
        n261 = disable-structure shown="Disabled" {
          disable-tunnel: w3276 -> [w3425 _]
          frame Disabled {
            n262 = call "FeedbackDecode_AllEMGHM.vi"("Intensities"=w3425, "Mode"=enum16{"Initialize", "Run"}."Run") -> ()  [unwired: 2 in]
          }
          frame Enabled {
          }
        }
        n263 = local write "NIPTime"(w3274) -> ()
        n264 = global write "FeedbackDecode_Globals.vi" "FD_NIPTime"(w3274) -> ()
        n265 = case shown="True" w3261 {
          tunnel: w3301 -> [_ w3413]
          frame False {
          }
          frame True {
            n266 = call-poly <vilib>:"DAQmx Write.vi"("task/channels in"=refnum<k21> "AO0", "data"=w3413) -> ()  [unwired: 11 in, 3 out]
          }
        }
        n267 = Array Subset(array=w3276, length=80) -> (w3277:dbl[])  [unwired: 1 in]
        n268 = Or Array Elements(Boolean array=w3264) -> (logical OR=w3263:bool)
        n269 = global read "FeedbackDecode_Globals.vi" "FD_AVIImage"() -> (→"AVIImage":T10)
        n270 = global read "FeedbackDecode_Globals.vi" "FD_FrameCount"() -> (→"FrameCount":i32)
        n271 = global read "FeedbackDecode_Globals.vi" "FD_SkippedFrames"() -> (→"SkippedFrames":i32)
        n272 = Build Array (concatenate)(w3340, w3277) -> (w3338:dbl[])
        n273 = call "FeedbackDecode_PtPtCorr.vi"("Rates"=w3338, "Initialize"="ResetCorr", "Training"=w3348, "Lag"=w3368) -> ("Corr"=w3367:dbl[])  [unwired: 1 in, 2 out]
        n274 = Reshape Array(w3367, 280.0 ("y"), w3369) -> (w3370:dbl[][])
        n275 = case shown="True" "HoldCorr" {
          tunnel: [w3484 w3485] -> w3337
          tunnel: w3370 -> [w3483 _]
          tunnel: w3364 -> [w3482 _]
          tunnel: w3363 -> [_ w3485]
          frame False {
            n276 = Index Array(array=w3483, index (col)=w3482) -> (element=w3484:dbl[])  [unwired: 1 in]
          }
          frame True {
          }
        }
        n277 = feedback-in #1(w3337) -> ()
        n278 = case shown="\"Rate\", Default" w3339 {
          tunnel: w3338 -> [w3475 _]
          tunnel: w3337 -> [_ w3477]
          tunnel: [w3475 w3477] -> w3324
          tunnel: ["HeatMap Range" cluster{"Min":dbl, "Max":dbl} {"Min"=0.0, "Max"=1.0} ("Range")] -> w3314
          frame "Rate", Default {
          }
          frame "Corr" {
          }
        }
        n279 = Array Subset(array=w3324, length=100) -> (w3321:dbl[])  [unwired: 1 in]
        n280 = Array Subset(array=w3324, index=100 ("length"), length=100) -> (w3320:dbl[])
        n281 = Array Subset(array=w3324, index=200 ("length"), length=80) -> (w3319:dbl[])
        n282 = Build Array(w3327, w3321, w3322) -> (w3326:dbl[][])
        n283 = Build Array(w3327, w3320, w3322) -> (w3325:dbl[][])
        n284 = Build Array(w3323, w3319, w3322) -> (w3318:dbl[][])
